vi "Colour to Greyscale.vi"(8 "error in (no error)":errorcluster, 11 "Colour":u32(colorbox)) -> (0 "error out":errorcluster, 3 "Grey":u32(colorbox))   [LabVIEW 2018, in "Colour Lab.lvlib"]
uses:
  Colour Lab.lvlib
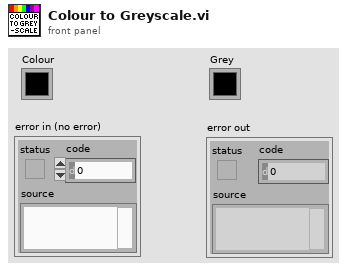
[diagram p1: front panel]
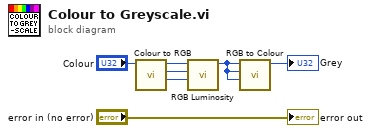
[diagram p0: block diagram]
diagram:
  n1 = call "Colour to RGB.vi"("Colour"="Colour") -> ("Blue"=w2:u8, "Green"=w3:u8, "Red"=w4:u8)  [unwired: 6 in, 2 out]
  n2 = call "RGB Luminosity.vi"("Blue"=w2, "Green"=w3, "Red"=w4) -> ("Luminosity"=w1:u8)  [unwired: 7 in, 1 out]
  n3 = call "RGB to Colour.vi"("Blue"=w1, "Green"=w1, "Red"=w1) -> ("Color"=→"Grey":u32)  [unwired: 7 in, 1 out]
  "error out" <- "error in (no error)"
